vi "UnlockDataFifo.vi"(8 "error in (no error)":errorcluster, 11 "PmuBase in":refnum<class "PmuBase.lvclass">) -> (0 "error out":errorcluster, 3 "PmuBase out":refnum<class "PmuBase.lvclass">)   [LabVIEW 2018, in "SensorPlugins.lvlib" / "PmuBase.lvclass"]
uses:
  PmuBase.lvclass
  PmuBase.lvclass/PmuBase.ctl
  Accessors/Read DataFifo.vi
  Accessors/Write DataFifo.vi
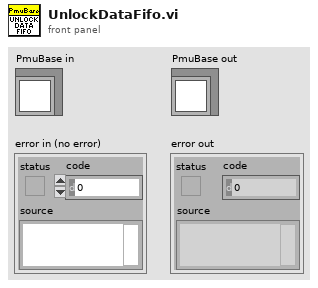
[diagram p1: front panel]
types:
  T1 = typedef "DataFifo.ctl" = cluster{"ReadPointer":u16, "WritePointer":u64, "Locked":bool, "FifoSize":u64}
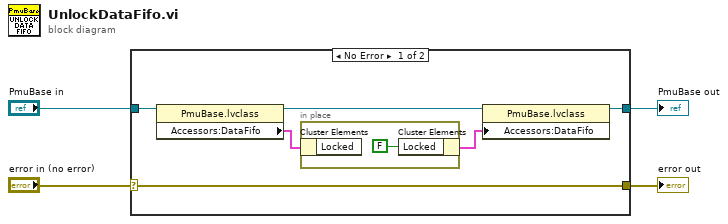
[diagram p0: block diagram]
diagram:
  n1 = case shown="No Error" "error in (no error)" {
    selector: "error in (no error)" -> [w9 w13]
    tunnel: [w9 w13] -> w3
    tunnel: [w7 w12] -> w1
    tunnel: "PmuBase in" -> [w10 w12]
    frame No Error {
      n2 = property class="PmuBase.lvclass"(reference=w10) -> (reference out=w8:refnum<class "PmuBase.lvclass">, "Accessors:DataFifo"=w6:T1)  [unwired: 1 in, 1 out]
      n3 = in-place {
        n4 = in-place-cluster #1(w6) -> ()  [unwired: 1 out]
        n5 = in-place-cluster #1("Locked"=FALSE) -> (w5:T1)
      }
      n6 = property class="PmuBase.lvclass"(reference=w8, "Accessors:DataFifo"=w5) -> (reference out=w7:refnum<class "PmuBase.lvclass">)  [unwired: 1 in, 1 out]
    }
    frame Error {
    }
  }
  "error out" <- w3
  "PmuBase out" <- w1
